vi "Display Error-Prompt.vi"(6 "Theme":refnum<class "Theme.lvclass">, 8 "error in":errorcluster, 10 "Error Message":string) -> (0 "error out":errorcluster, 1 "Choice?":bool)   [LabVIEW 2021, in "Pop-Up.lvlib" / "Error-Prompt.lvclass"]
doc: "This VI shows a common error prompt dialog.\n\n<b>Code Developed By:</b> +\nDaniel Coons +\nhttps://github.com/danielcoons/tsc-pop-up"
uses:
  Error-Prompt.lvclass
  Theme/Theme.lvclass
  C:/Development/Open Source/tsc-pop-up/Popup/Popup.lvclass
  Popup/Data Member Access/Write Theme.vi
  Error-Prompt.lvclass/Error-Prompt.ctl
  Popup/Popup.lvclass
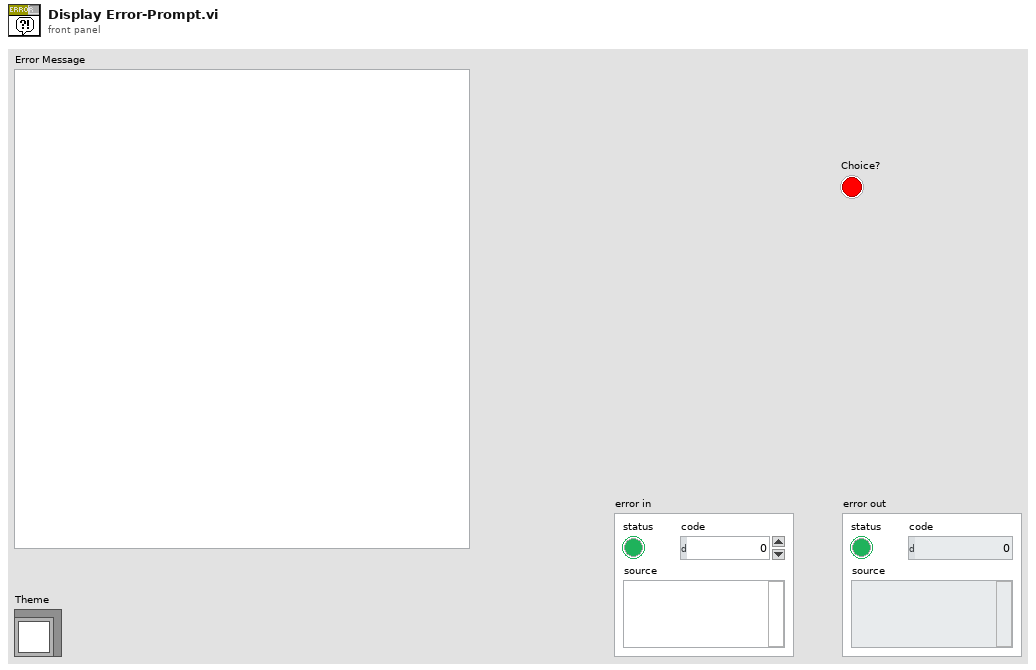
[diagram p1: front panel]
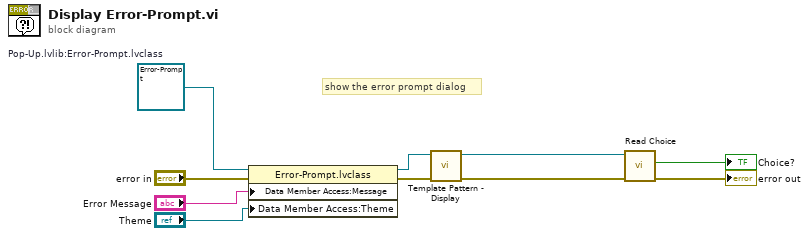
[diagram p0: block diagram]
diagram:
  w9 = refnum<class "Error-Prompt.lvclass"> refnum  # Pop-Up.lvlib:Error-Prompt.lvclass
  # "show the error prompt dialog"
  n1 = property on="Property Node" class="Error-Prompt.lvclass"(reference=w9, error in="error in", "Data Member Access:Message"="Error Message", "Data Member Access:Theme"="Theme") -> (reference out=w4:refnum<class "Error-Prompt.lvclass">, error out=w5:errorcluster)
  n2 = call "Template Pattern - Display.vi"("error in (no error)"=w5, "PopUp in"=w4) -> ("error out"=w3:errorcluster, "PopUp out"=w6:refnum<class "Error-Prompt.lvclass">)  [unwired: 8 in]
  n3 = call-dynamic "Read Choice.vi"("error in (no error)"=w3, "_Popup in"=w6) -> ("error out"=→"error out":errorcluster, "Choice"=→"Choice?":bool)  [unwired: 7 in, 1 out]
